vi "Magazine_Notifier_Begin.vi"   [LabVIEW 2020]
uses:
  Subsystems/Arrow/Magazine_Cluster.ctl
  Subsystems/Arrow/Magazine_Control_States.ctl
  Globals/Magazine_Globals.vi
types:
  T1 = typedef "Magazine_Cluster.ctl" = cluster{"Control_States":T2, "Manual_Magazine":dbl, "GoToAngle":bool}
  T2 = typedef "Magazine_Control_States.ctl" = enum16{"No-Op", "Manual_Control", "Load", "Firing"}
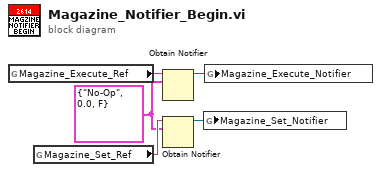
[diagram p0: block diagram]
diagram:
  w1 = T1 {"Control_States"=enum."No-Op", "Manual_Magazine"=0.0, "GoToAngle"=FALSE}
  n1 = global read "Magazine_Globals.vi" "Magazine_Execute_Ref"() -> (w2:string)
  n2 = global read "Magazine_Globals.vi" "Magazine_Set_Ref"() -> (w3:string)
  n3 = Obtain Notifier(name (unnamed)=w2, notification data type=w1) -> (notifier out=w5:refnum<notifier>)  [unwired: 2 in, 2 out]
  n4 = Obtain Notifier(name (unnamed)=w3, notification data type=w1) -> (notifier out=w4:refnum<notifier>)  [unwired: 2 in, 2 out]
  n5 = global write "Magazine_Globals.vi" "Magazine_Set_Notifier"(w4) -> ()
  n6 = global write "Magazine_Globals.vi" "Magazine_Execute_Notifier"(w5) -> ()
